vi "IB_ReadLog (Inside).vi"() -> (6 "Array":dbl[](array[numeric]))   [LabVIEW 2013]
panel:
  out "Temperature (C, D, E, F)":string[](array[string])
  out "F":cluster{timestamp[], dbl[]}(graph)
  out "E":cluster{timestamp[], dbl[]}(graph)
  out "D":cluster{timestamp[], dbl[]}(graph)
  out "C":cluster{timestamp[], dbl[]}(graph)
  out "Time Stamp":timestamp[](array[timestamp])
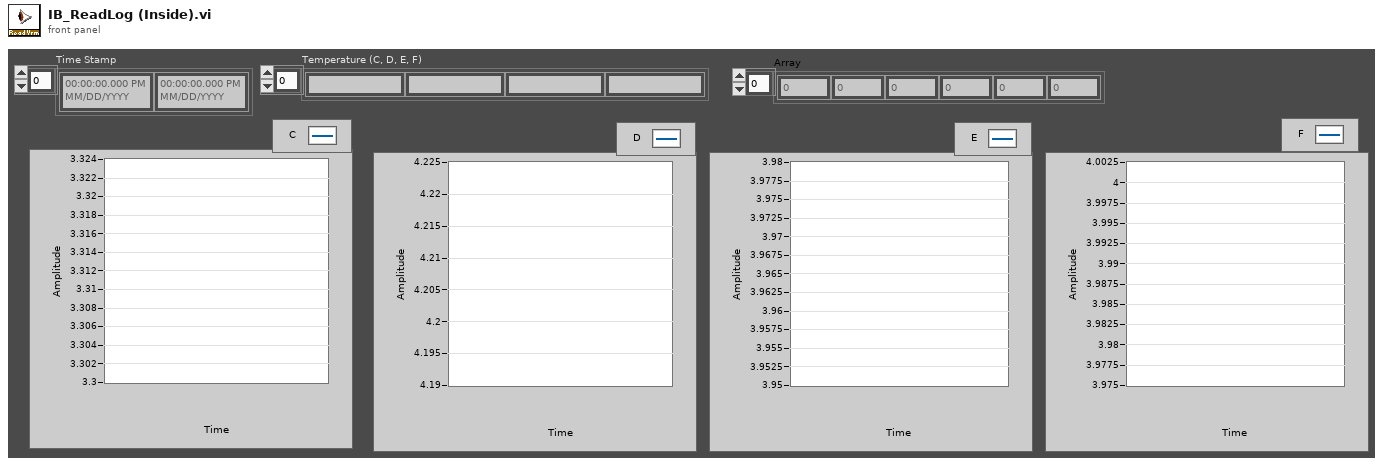
[diagram p1: front panel]
types:
  T1 = cluster{"second":i32, "minute":i32, "hour":i32, "day of month":i32, "month":i32, "year":i32, "day of week":i32, "day of year":i32, "is DST":i32}
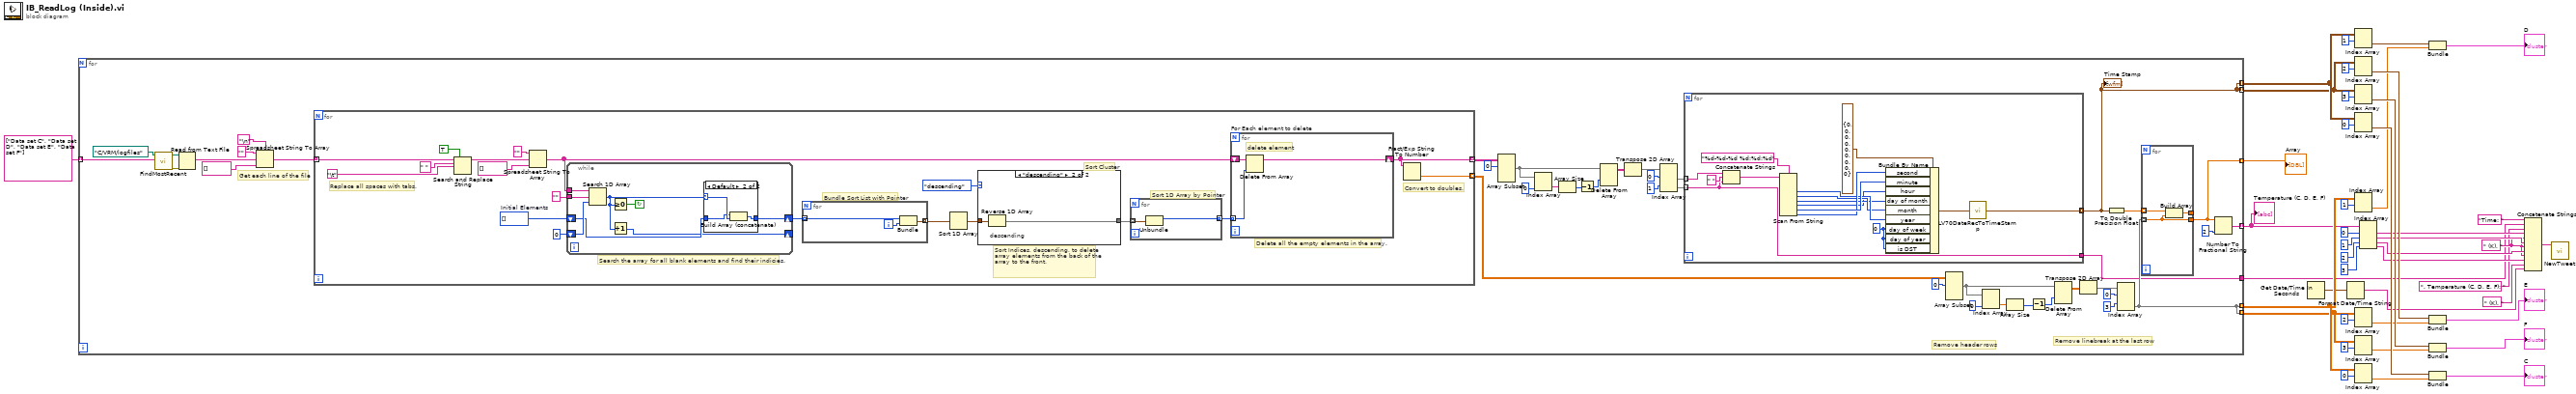
[diagram p0: block diagram]
diagram:
  w10 = " (K), " ("string")
  n1 = for {
    tunnel: string[] ["Data set C", "Data set D", "Data set E", "Data set F"] -> [w50] mode=indexing
    tunnel: [w49] -> w36 mode=indexing
    tunnel: [w48] -> w35 mode=indexing
    tunnel: [w49] -> w30 mode=indexing
    tunnel: [w48] -> w29 mode=indexing
    tunnel: [w47] -> w18 mode=indexing
    tunnel: [w45] -> w6
    tunnel: [w44] -> w1 mode=indexing
    # "Remove linebreak at the last row"
    # "Remove header rows"
    # "Get each line of the file"
    n2 = call "FindMostRecent.vi"("Filename Pattern"=w50, "Folder Path In"=path "C:/VRM/logfiles") -> ("error out"=w51:errorcluster, "File Path for the Newest File"=w52:path)  [unwired: 8 in]
    n3 = Read from Text File(file (use dialog)=w52, error in=w51) -> (text=w83:string)  [unwired: 5 out]
    n4 = Spreadsheet String To Array(delimiter (Tab)="\n", format string="", spreadsheet string=w83, array type (2D Dbl)=string[] []) -> (array=w79:string[])
    n5 = for {
      tunnel: w79 -> [w120] mode=indexing
      tunnel: [w102] -> w61 mode=indexing
      tunnel: [w103] -> w75 mode=indexing
      w112 = i32[] []  # Initial Elements
      # "Convert to doubles."
      # "Delete all the empty elements in the array."
      # "Search the array for all blank elements and find their indicies."
      # "Replace all spaces with tabs."
      # "Sort 1D Array by Pointer"
      # "Sort Cluster"
      # "Bundle Sort List with Pointer"
      # "Sort Indices, descending, to delete array elements from the back of the array to the front."
      n6 = Search and Replace String(replace all?=TRUE ("replace all? (F)"), input string=w120, search string=" ", replace string="\t") -> (result string=w115:string)  [unwired: 1 in, 6 out]
      n7 = Spreadsheet String To Array(format string="", spreadsheet string=w115, array type (2D Dbl)=string[] []) -> (array=w110:string[])  [unwired: 1 out]
      n8 = while {
        shift-right: [w132] -> _
        shift-left: 0 -> [w139]
        shift-right: [w136] -> w106
        shift-left: w112 -> [w137]
        tunnel: w110 -> [w138]
        tunnel: "" ("Element Data") -> [w135]
        stop <- w133 continue-if-true
        n9 = Search 1D Array(1D array=w138, element=w135, start index (0)=w139) -> (index of element=w134:i32)
        n10 = Greater Or Equal To 0?(x=w134) -> (x >= 0?=w133:bool)
        n11 = Increment(x=w134) -> (x+1=w132:i32)
        n12 = case shown="Default" w134 {
          selector: w134 -> [_ w143]
          tunnel: w137 -> [w140 w142]
          tunnel: [w140 w141] -> w136
          frame -1 {
          }
          frame Default {
            n13 = Build Array (concatenate)(w142, w143) -> (w141:i32[])
          }
        }
      }
      n14 = for {
        tunnel: w106 -> [w123] mode=indexing
        tunnel: [w121] -> w108 mode=indexing
        i -> [w122]
        n15 = Bundle("index of element"=w123, w122) -> (w121:cluster{"index of element":i32, i32})  [unwired: 1 out]
      }
      n16 = Sort 1D Array(array=w108) -> (sorted array=w107:cluster{"index of element":i32, i32}[])
      n17 = case shown="\"descending\"" enum16{"ascending", "descending"}."descending" ("Order") {
        tunnel: [w124 w125] -> w109
        tunnel: w107 -> [w124 w126]
        frame "ascending", Default {
        }
        frame "descending" {
          # "descending"
          n18 = Reverse 1D Array(array=w126) -> (reversed array=w125:cluster{"index of element":i32, i32}[])
        }
      }
      n19 = for {
        tunnel: w109 -> [w128] mode=indexing
        tunnel: [w127] -> w104 mode=indexing
        n20 = Unbundle(w128) -> ("index of element"=w127:i32)  [unwired: 1 out]
      }
      n21 = for "For Each element to delete" {
        tunnel: w104 -> [w131] mode=indexing
        shift-right: [w130] -> w102
        shift-left: w110 -> [w129]
        # "delete element"
        n22 = Delete From Array(array=w129, index=w131) -> (array with subset deleted=w130:string[])  [unwired: 1 in, 1 out]
      }
      n23 = Fract/Exp String To Number(string=w102) -> (number=w103:dbl[])  [unwired: 4 out]
    }
    n24 = Array Subset(array=w61, index (row)=0 ("index")) -> (w62:string[][])  [unwired: 3 in]
    n25 = Index Array(array=w62, index (col)=0 ("disabled index (col)")) -> (element=w65:string[])  [unwired: 1 in]
    n26 = Array Size(array=w65) -> (size(s)=w64:i32)
    n27 = Decrement(x=w64) -> (x-1=w63:i32)
    n28 = Delete From Array(array=w62, index (row)=w63) -> (array with subset deleted=w60:string[][])  [unwired: 2 in, 1 out]
    n29 = Transpose 2D Array(2D array=w60) -> (transposed array=w57:string[][])
    n30 = Index Array(array=w57, index (row) #1=0 ("disabled index (col)"), index (row) #2=1 ("index (col)")) -> (element #1=w56:string[], element #2=w55:string[])  [unwired: 2 in]
    n31 = for {
      tunnel: w56 -> [w97] mode=indexing
      tunnel: w55 -> [w84] mode=indexing
      tunnel: [w85] -> w49 mode=indexing
      tunnel: [w84] -> w45
      w94 = 0
      n32 = Concatenate Strings(w97, " " ("string"), w84) -> (w86:string)
      n33 = Scan From String "Scan From String"(format string="%d-%d-%d %d:%d:%d", input string=w86) -> (output 1=w91:i32, output 2=w90:i32, output 3=w89:i32, output 4=w88:i32, output 5=w93:i32, output 6=w92:i32)  [unwired: 8 in, 3 out]
      n34 = Bundle By Name(cluster=T1 {"second"=0, "minute"=0, "hour"=0, "day of month"=0, "month"=0, "year"=0, "day of week"=0, "day of year"=0, "is DST"=0} ("date time rec"), "second"=w92, "minute"=w93, "hour"=w88, "day of month"=w89, "month"=w90, "year"=w91, "day of week"=w94, "day of year"=w94, "is DST"=w94) -> (w95:T1)
      n35 = call <vilib>:"LV70DateRecToTimeStamp.vi"("date time rec"=w95) -> ("Time Stamp"=w85:timestamp)
    }
    "Time Stamp" <- w49
    n36 = Array Subset(array=w75, index (row)=0 ("index")) -> (w69:dbl[][])  [unwired: 3 in]
    n37 = Index Array(array=w69, index (col)=0 ("disabled index (col)")) -> (element=w73:dbl[])  [unwired: 1 in]
    n38 = Array Size(array=w73) -> (size(s)=w71:i32)
    n39 = Decrement(x=w71) -> (x-1=w70:i32)
    n40 = Delete From Array(array=w69, index (row)=w70) -> (array with subset deleted=w72:dbl[][])  [unwired: 2 in, 1 out]
    n41 = Transpose 2D Array(2D array=w72) -> (transposed array=w68:dbl[][])
    n42 = To Double Precision Float(number=w49) -> (double precision float=w54:dbl[])
    n43 = Index Array(array=w68, index (row) #1=0 ("index (row)"), index (row) #2=3 ("index (row)")) -> (element #2=w48:dbl[])  [unwired: 2 in, 1 out]
    n44 = for {
      tunnel: w48 -> [w99] mode=indexing
      tunnel: [w101] -> _
      tunnel: w54 -> [w100] mode=indexing
      tunnel: [w99] -> w44
      n45 = Build Array(w100, w99) -> (w101:dbl[])
    }
    n46 = Number To Fractional String(number=w44, precision (6)=i16 2 ("width (-)")) -> (F-format string=w47:string)  [unwired: 2 in]
  }
  "Temperature (C, D, E, F)" <- w18
  "Array" <- w1
  n47 = Get Date/Time In Seconds() -> (seconds since 1Jan1904=w3:timestamp)
  n48 = Format Date/Time String(seconds (now)=w3) -> (date/time string=w2:string)  [unwired: 2 in]
  n49 = Index Array(array=w35, index (row)=1) -> (element=w23:dbl[])  [unwired: 1 in]
  n50 = Index Array(array=w29, index (row)=2) -> (element=w25:dbl[])  [unwired: 1 in]
  n51 = Index Array(array=w29, index (row)=3) -> (element=w27:dbl[])  [unwired: 1 in]
  n52 = Index Array(array=w35, index (row)=0) -> (element=w39:dbl[])  [unwired: 1 in]
  n53 = Index Array(array=w36, index (row)=1) -> (element=w24:timestamp[])  [unwired: 1 in]
  n54 = Index Array(array=w30, index (row)=2) -> (element=w26:timestamp[])  [unwired: 1 in]
  n55 = Index Array(array=w30, index (row)=3) -> (element=w28:timestamp[])  [unwired: 1 in]
  n56 = Index Array(array=w36, index (row)=0) -> (element=w41:timestamp[])  [unwired: 1 in]
  n57 = Index Array(array=w18, index #1=0 ("index"), index #2=1 ("index"), index #3=2 ("index"), index #4=3 ("index")) -> (element #1=w13:string, element #2=w12:string, element #3=w11:string, element #4=w9:string)
  n58 = Bundle(w24, w23) -> (→"D":cluster{timestamp[], dbl[]})  [unwired: 1 in]
  n59 = Bundle(w26, w25) -> (→"E":cluster{timestamp[], dbl[]})  [unwired: 1 in]
  n60 = Bundle(w28, w27) -> (→"F":cluster{timestamp[], dbl[]})  [unwired: 1 in]
  n61 = Bundle(w41, w39) -> (→"C":cluster{timestamp[], dbl[]})  [unwired: 1 in]
  n62 = Concatenate Strings("Time: " ("string"), w6, ". Temperature (C, D, E, F): " ("string"), w13, w10, w12, w10, w11, w10, w9, " (K). " ("string"), w2) -> (w8:string)
  n63 = call "NewTweet.vi"("Message Main Body"=w8) -> ()  [unwired: 11 in]
